vi "stop_program.vi"(2 "filename":refnum<file>, 3 "VISA resource name":refnum<visa-resource-name>, 4 "error in (no error)":errorcluster, 5 "stop":bool, 6 "Run Info Cluster In":T1={"Set Point (*C)"=0, "Field (uT)"=0.0, "Soak Time (min)"=30, "Field on/off"=FALSE, "Atmosphere"="1", "Use DB"=enum."DB Yes", "User ID"="", "Batch / Boat ID"="", "User"="", "Note"="", "Field on (C)"=0.0, "Field off (C)"=0.0, "email address"="", "Control ramp"=FALSE, "Ramp rate"=1.0, "Contact Me"=enum."E-mail", "Test e-mail"=FALSE, "Cellular Provider"=""} {"Ramp rate" min=1.0 max=100.0}, 7 "Datafile blob":string) -> (0 "error out":errorcluster, 1 "Reset?":bool)   [LabVIEW 2009]
doc: "Prompts user to confirm quit, then closes datafile and stops vi execution"
panel:
  # "Run Information"
  # "(deg/min)"
  # "E-mail or text me when done at:"
  # "(enter e-mail address or phone number)"
  # "User Information"
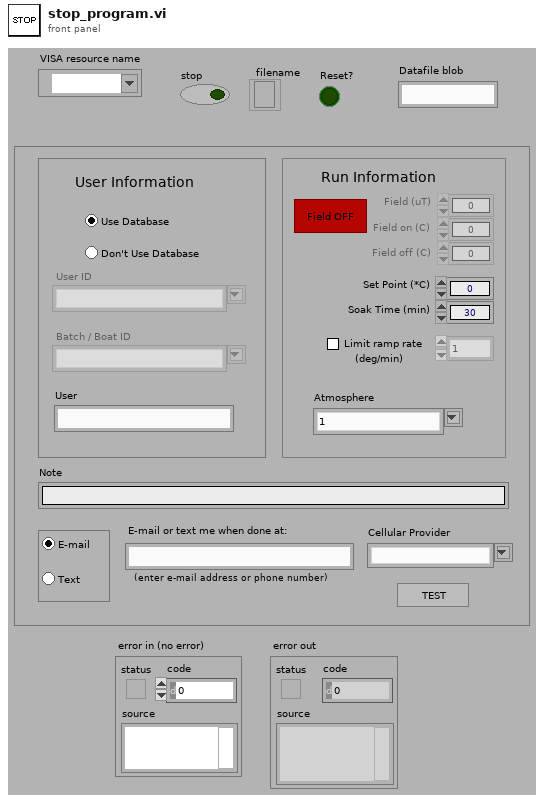
[diagram p1: front panel]
types:
  T1 = cluster{"Set Point (*C)":u32, "Field (uT)":dbl, "Soak Time (min)":u32, "Field on/off":bool, "Atmosphere":string, "Use DB":enum32{"DB Yes", "DB no"}, "User ID":string, "Batch / Boat ID":string, "User":string, "Note":string, "Field on (C)":dbl, "Field off (C)":dbl, "email address":string, "Control ramp":bool, "Ramp rate":dbl, "Contact Me":enum32{"No Selection", "E-mail", "Text"}, "Test e-mail":bool, "Cellular Provider":string}
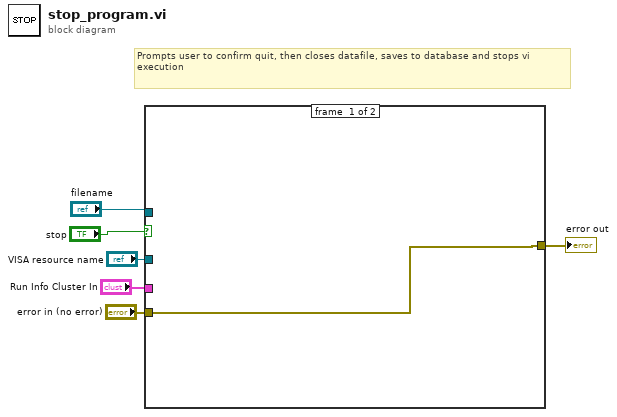
[diagram p0: block diagram]
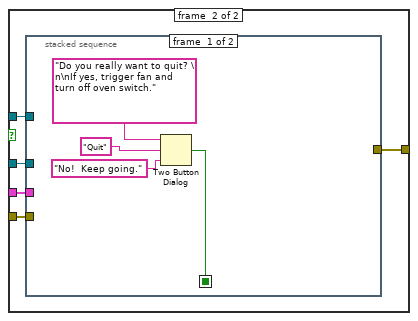
[diagram p2: hidden frame]
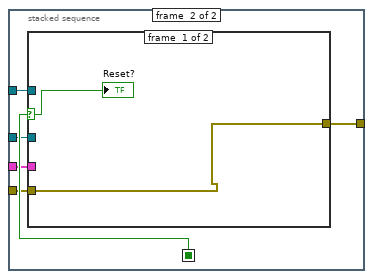
[diagram p3: hidden frame]
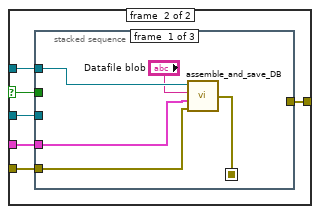
[diagram p4: hidden frame]
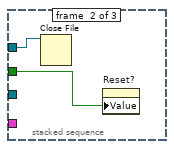
[diagram p5: hidden frame]
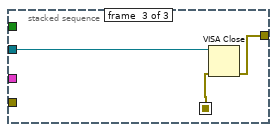
[diagram p6: hidden frame]
diagram:
  # "Prompts user to confirm quit, then closes datafile, saves to database and stops vi execution"
  n1 = case shown="True" "stop" {
    tunnel: "filename" -> [_ w12]
    tunnel: "Run Info Cluster In" -> [_ w11]
    tunnel: "error in (no error)" -> [w7 w10]
    tunnel: [w7 w9] -> w3
    tunnel: "VISA resource name" -> [_ w8]
    frame #0 {
    }
    frame #1 {
      n2 = stacked-sequence {
        seq-local: [w13 _] -> [_ w22]
        tunnel: w12 -> [_ w21]
        tunnel: w11 -> [_ w20]
        tunnel: w10 -> [_ w19]
        tunnel: [_ w18] -> w9
        tunnel: w8 -> [_ w17]
        frame #0 {
          n3 = Two Button Dialog(message="Do you really want to quit? \n\nIf yes, trigger fan and turn off oven switch.", 1:"No!  Keep going.", 2:"Quit") -> (T button?=w13:bool)
        }
        frame #1 {
          n4 = case shown="True" w22 {
            selector: w22 -> [w24 w29]
            tunnel: w21 -> [_ w30]
            tunnel: w20 -> [_ w28]
            tunnel: w19 -> [w23 w27]
            tunnel: [w23 w26] -> w18
            tunnel: w17 -> [_ w25]
            frame #0 {
              "Reset?" <- w24
            }
            frame #1 {
              n5 = stacked-sequence {
                seq-local: [w32 _ _] -> [_ _ w39]
                tunnel: w30 -> [w35 w37 _]
                tunnel: w29 -> [_ w36 _]
                tunnel: w28 -> [w31 _ _]
                tunnel: w27 -> [w33 _ _]
                tunnel: [_ _ w38] -> w26
                tunnel: w25 -> [_ _ w40]
                frame #0 {
                  n6 = call "assemble_and_save_DB.vi"("error in (no error)"=w33, "Run Info Cluster In"=w31, "Datafile blob"="Datafile blob", "filename"=w35) -> ("error out"=w32:errorcluster)
                }
                frame #1 {
                  n7 = Close File(refnum=w37) -> ()  [unwired: 1 in, 2 out]
                  n8 = property on="Reset?" class="Bool (strict)"("Value"=w36) -> ()  [unwired: 2 in, 2 out]
                }
                frame #2 {
                  n9 = VISA Close(VISA resource name=w40, error in (no error)=w39) -> (error out=w38:errorcluster)
                }
              }
            }
          }
        }
      }
    }
  }
  "error out" <- w3
